vi "Get Magnet.vi"(6 "Axis":T1, 8 "error in (no error)":errorcluster, 11 "Instrument.VRM in":refnum<class "Instrument.OxfordVRM.lvclass">) -> (0 "error out":errorcluster, 1 "Status":string, 2 "B Field (T)":dbl, 3 "Instrument.VRM out":refnum<class "Instrument.OxfordVRM.lvclass">, 4 "Finished?":bool)   [LabVIEW 2019, in "Instrument.OxfordVRM.lvclass"]
uses:
  Instrument.OxfordVRM.lvclass
  73b42b6d-ba68-499e-af67-1842dcc5431a.vi
  Typedefs/Instrument.VRM.publicCommands-enum.ctl
  Typedefs/VRM Magnet Axis--Enum.ctl
  Typedefs/Instrument.VRM.getMagnetRequest--cluster.ctl
  Typedefs/Instrument.VRM.getMagnet-cluster.ctl
  <userlib>/LevyLab/Instrument Framework/Instrument Types/Cryostat/Typedefs/Magnet Axis--Enum.ctl
  <userlib>/LevyLab/Instrument Framework/Instrument Types/Cryostat/Instrument.Cryostat.lvclass
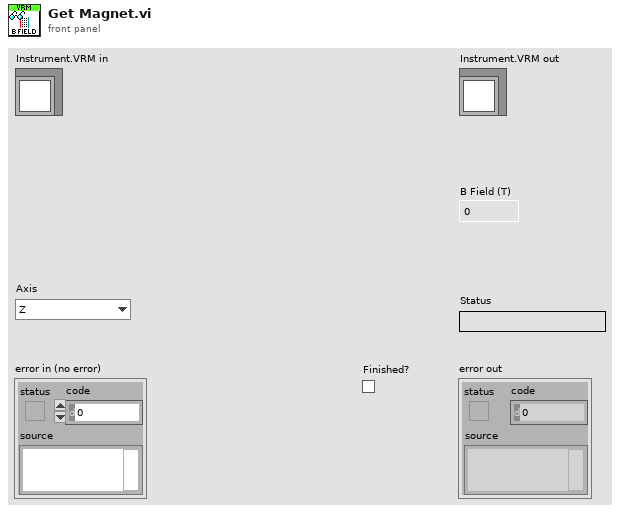
[diagram p1: front panel]
types:
  T1 = typedef "Instrument.Cryostat.lvclass/Magnet Axis--Enum.ctl" = enum16{"Z", "X", "Y"}
  T2 = typedef "Instrument.OxfordVRM.lvclass/Instrument.VRM.getMagnet-cluster.ctl" = cluster{"field":dbl, "status":string, "finished":bool}
  T3 = typedef "Instrument.OxfordVRM.lvclass/Instrument.VRM.getMagnetRequest--cluster.ctl" = cluster{"Axis":T4}
  T4 = typedef "Instrument.OxfordVRM.lvclass/VRM Magnet Axis--Enum.ctl" = enum16{"Z", "X", "Y", "ALL"}
  T5 = typedef "Instrument.OxfordVRM.lvclass/Instrument.VRM.publicCommands-enum.ctl" = enum16{"setMagnet", "getMagnet"}
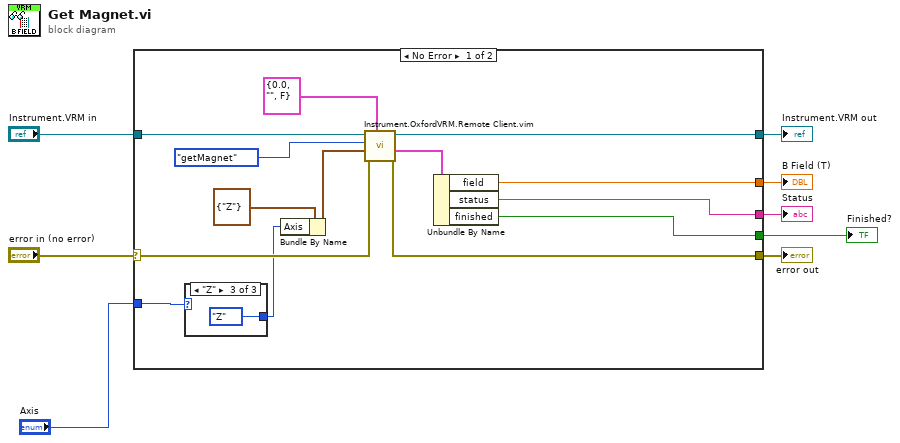
[diagram p0: block diagram]
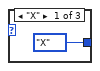
[diagram p2: hidden frame]
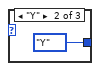
[diagram p3: hidden frame]
diagram:
  n1 = case shown="No Error" "error in (no error)" {
    selector: "error in (no error)" -> [w21 w27]
    tunnel: "Instrument.VRM in" -> [w22 w26]
    tunnel: [w18 w26] -> w7
    tunnel: [w12 _] -> w6
    tunnel: [w9 w27] -> w4
    tunnel: [w11 _] -> w3
    tunnel: "Axis" -> [w19 _]
    tunnel: [w10 _] -> w1
    frame No Error {
      n2 = case shown="\"Z\"" w19 {
        tunnel: [VRM_Magnet_Axis--Enum."X" ("Target.Axis") VRM_Magnet_Axis--Enum."Y" ("Target.Axis") VRM_Magnet_Axis--Enum."Z" ("Target.Axis")] -> w16
        frame "X" {
        }
        frame "Y" {
        }
        frame "Z" {
        }
      }
      n3 = Bundle By Name(cluster=T3 {"Axis"=enum."Z"} ("getMagnetRequest"), "Axis"=w16) -> (w15:T3)
      n4 = call "Instrument.OxfordVRM.Remote Client.vim"("Data Out type"=T2 {"field"=0.0, "status"="", "finished"=FALSE} ("getMagnet"), "error in (no error)"=w21, "Data"=w15, "Commands"=Instrument.VRM.publicCommands-enum."getMagnet", "Instrument.VRM in"=w22) -> ("error out"=w9:errorcluster, "Data out"=w13:T2, "Instrument.VRM out"=w18:refnum<class "Instrument.OxfordVRM.lvclass">)  [unwired: 4 in]
      n5 = Unbundle By Name(w13) -> ("field"=w12:dbl, "status"=w11:string, "finished"=w10:bool)
    }
    frame Error {
    }
  }
  "error out" <- w4
  "Instrument.VRM out" <- w7
  "B Field (T)" <- w6
  "Status" <- w3
  "Finished?" <- w1
